vi "instantiate_weviate_vector.vi"(0 "host_url":string, 5 "api_key":string, 11 "error in":errorcluster) -> (4 "vector_weviate.lvclass":refnum<class "vector_weviate.lvclass">, 15 "error out":errorcluster)   [LabVIEW 2020, in "vector_weviate.lvclass"]
uses:
  vector_weviate.lvclass
  vector_weviate.lvclass/vector_weviate.ctl
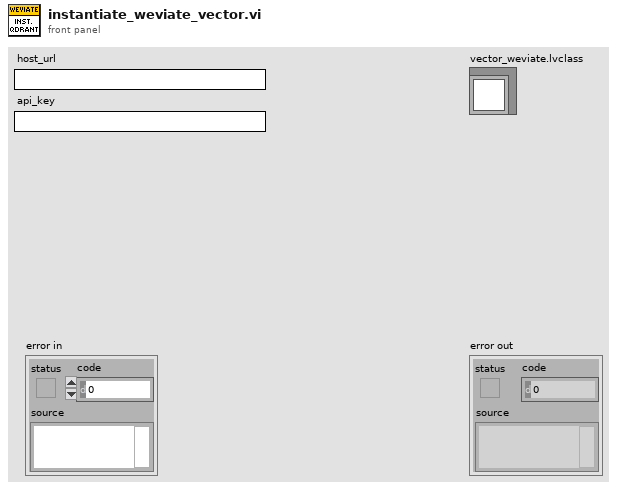
[diagram p1: front panel]
types:
  T1 = typedef "LabVIEWHTTPClient.lvlib/ClientHandle.ctl" = refnum<k1>
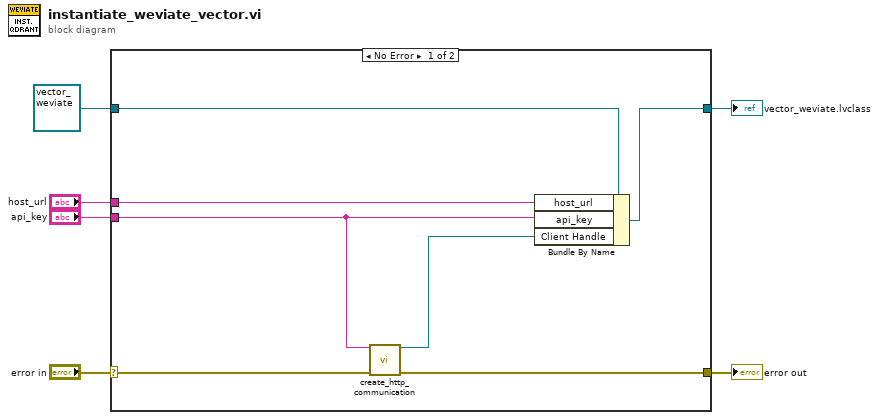
[diagram p0: block diagram]
diagram:
  n1 = case shown="No Error" "error in" {
    selector: "error in" -> [w12 w15]
    tunnel: [w11 w15] -> w5
    tunnel: [w7 w14] -> w1
    tunnel: refnum<class "vector_weviate.lvclass"> refnum ("vector_weviate.lvclass") -> [w8 w14]
    tunnel: "host_url" -> [w13 _]
    tunnel: "api_key" -> [w10 _]
    frame No Error {
      n2 = call "create_http_communication.vi"("api_key"=w10, "error in"=w12) -> ("client handle"=w9:T1, "error out"=w11:errorcluster)  [unwired: 12 in]
      n3 = Bundle By Name(cluster=w8, "host_url"=w13, "api_key"=w10, "Client Handle"=w9) -> (w7:refnum<class "vector_weviate.lvclass">)
    }
    frame Error {
    }
  }
  "error out" <- w5
  "vector_weviate.lvclass" <- w1
